vi "Write A-V and Publish.vi"(6 "measurement":dbl format="%^.2e", 8 "error in (no error)":errorcluster, 9 "measurement type (voltage)":i32(ring)=1 items=["Voltage"=1, "Current"=0], 10 "channel name (\"CHANNEL1\")":string="CHANNEL1", 11 "CS++DCPwr in":refnum<class "CS++DCPwr.lvclass">) -> (0 "error out":errorcluster, 3 "CS++DCPwr out":refnum<class "CS++DCPwr.lvclass">)   [LabVIEW 2015, in "CS++DCPwr.lvlib" / "CS++DCPwr.lvclass"]
doc: "Write measurement value to attribute and publish to PV."
uses:
  CS++DCPwr.lvclass
  CSPP_Core/Classes/CS++ProcessVariables/ProcessVariable/PV.lvclass
  CS++DCPwr.lvclass/CS++DCPwr.ctl
  PV-Enum.ctl
  CSPP_Core/Classes/CS++ProcessVariables/ProcessVariable/PV.lvclass/PV.ctl
  CSPP_Core/Classes/CS++ProcessVariables/ProcessVariable/Write Data.vi
  CSPP_Core/Classes/CS++ProcessVariables/ProcessVariable/Write Timestamp.vi
  CSPP_Core/Classes/CS++ProcessVariables/ProcessVariable/Write Error.vi
  CSPP_Core/Classes/CS++ProcessVariables/PVConnection/PVConnection.lvclass
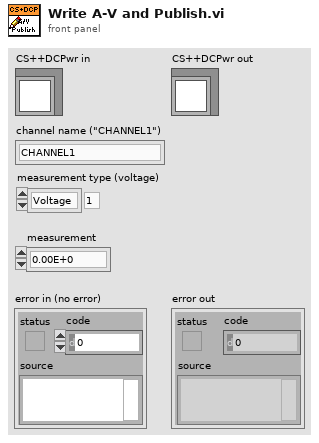
[diagram p1: front panel]
types:
  T1 = typedef "CS++DCPwr.lvlib/CS++DCPwr.lvclass/PV-Enum.ctl" = enum16{"CurrentLimit", "MaxCurrentLimit", "MaxVoltageLevel", "Measure-A", "Measure-V", "OVPLimit", "Range", "TriggerCurrentLimit", "TriggerVoltageLevel", "VoltageLevel", "Behavior", "DesiredOutputState", "RangeType", "TriggerSource", "InState", "OutputEnable", "OVPEnabled"}
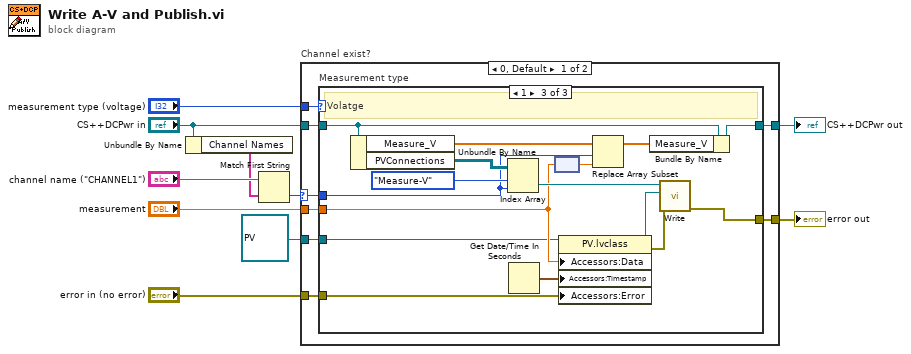
[diagram p0: block diagram]
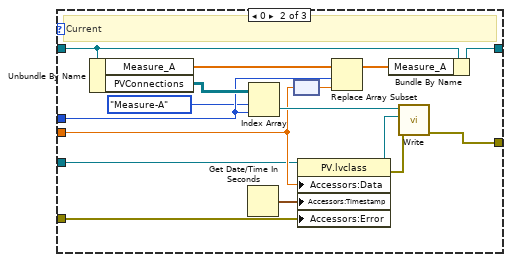
[diagram p3: hidden frame]
diagram:
  n1 = Unbundle By Name("CS++DCPwr in") -> ("Channel Names"=w6:string[])
  n2 = Match First String(2:w6, 3:"channel name (\"CHANNEL1\")") -> (0:w5:i32)  [unwired: 1 out]
  n3 = case "Channel exist?" shown="0, Default" w5 {
    selector: w5 -> [w14 _]
    tunnel: [w17 w54] -> w9
    tunnel: "CS++DCPwr in" -> [w16 w54]
    tunnel: "measurement type (voltage)" -> [w18 _]
    tunnel: "measurement" -> [w15 _]
    tunnel: "error in (no error)" -> [w13 w53]
    tunnel: [w12 w53] -> w3
    tunnel: refnum<class "PV.lvclass"> refnum ("PV") -> [w11 _]
    frame 0, Default {
      n4 = case "Measurement type" shown="1" w18 {
        tunnel: [w20 w35 w51] -> w17
        tunnel: w16 -> [w20 w36 w52]
        tunnel: w15 -> [_ w28 w44]
        tunnel: w14 -> [_ w22 w37]
        tunnel: w13 -> [w19 w25 w41]
        tunnel: [w19 w24 w40] -> w12
        tunnel: w11 -> [_ w23 w39]
        frame Default {
        }
        frame 0 {
          # "Current"
          n5 = Unbundle By Name(w36) -> ("Measure_A"=w34:dbl[unit][], "PVConnections"=w31:refnum<class "PVConnection.lvclass">[][])
          n6 = Get Date/Time In Seconds() -> (seconds since 1Jan1904=w26:timestamp)
          n7 = Index Array(array=w31, index (row)=PV-Enum."Measure-A" ("PV-Enum"), index (col)=w22) -> (element=w30:refnum<class "PVConnection.lvclass">)
          n8 = node(w28) -> (w32:dbl[unit])
          n9 = property class="PV.lvclass"(reference=w23, "Accessors:Data"=w28, "Accessors:Timestamp"=w26, "Accessors:Error"=w25) -> (reference out=w29:refnum<class "PV.lvclass">, error out=w27:errorcluster)  [unwired: 1 in]
          n10 = Replace Array Subset(array=w34, new element=w32, index=w22) -> (w33:dbl[unit][])
          n11 = Bundle By Name(cluster=w36, "Measure_A"=w33) -> (w35:refnum<class "CS++DCPwr.lvclass">)
          n12 = call "Write.vi"("error in (no error)"=w27, "PV"=w29, "PVConnection in"=w30) -> ("error out"=w24:errorcluster)  [unwired: 7 in, 1 out]
        }
        frame 1 {
          # "Volatge"
          n13 = Unbundle By Name(w52) -> ("Measure_V"=w50:dbl[unit][], "PVConnections"=w47:refnum<class "PVConnection.lvclass">[][])
          n14 = Index Array(array=w47, index (row)=PV-Enum."Measure-V" ("PV-Enum"), index (col)=w37) -> (element=w46:refnum<class "PVConnection.lvclass">)
          n15 = Get Date/Time In Seconds() -> (seconds since 1Jan1904=w42:timestamp)
          n16 = node(w44) -> (w48:dbl[unit])
          n17 = property class="PV.lvclass"(reference=w39, "Accessors:Data"=w44, "Accessors:Timestamp"=w42, "Accessors:Error"=w41) -> (reference out=w45:refnum<class "PV.lvclass">, error out=w43:errorcluster)  [unwired: 1 in]
          n18 = Replace Array Subset(array=w50, new element=w48, index=w37) -> (w49:dbl[unit][])
          n19 = Bundle By Name(cluster=w52, "Measure_V"=w49) -> (w51:refnum<class "CS++DCPwr.lvclass">)
          n20 = call "Write.vi"("error in (no error)"=w43, "PV"=w45, "PVConnection in"=w46) -> ("error out"=w40:errorcluster)  [unwired: 7 in, 1 out]
        }
      }
    }
    frame -1 {
    }
  }
  "error out" <- w3
  "CS++DCPwr out" <- w9
